vi "Gergberg Main.vi"() -> ()   [LabVIEW 2012, in "LightPipes.lvlib"]
uses:
  LightPipes.lvlib
panel:
  out "n_grid":i32=400
  in  "Number of Iteration":i32=20
  in  "MF Crop Size":i32=1000
  out "MF Interp Size":cluster{"x":i32, "y":i32}={"x"=1000, "y"=1000}
  out "MF Interped Pic":T1(plugin-control)
  in  "MF Interp Ratio":dbl=1.0
  in  "Mid Field":path=path "E:/MidfieldFarfieldForAaron/005778 2013-02-12/OSP Midfield.png"
  out "FF Interp Size":cluster{"x":i32, "y":i32}={"x"=1000, "y"=1000}
  out "FF Interp Pic":T1(plugin-control)
  in  "FF Crop Size":i32=400
  in  "FF Interp Ratio":dbl=2.5
  in  "Far Field":path=path "E:/MidfieldFarfieldForAaron/005778 2013-02-12/OSP FF.png"
  # "Far Field"
  # "Mid Field"
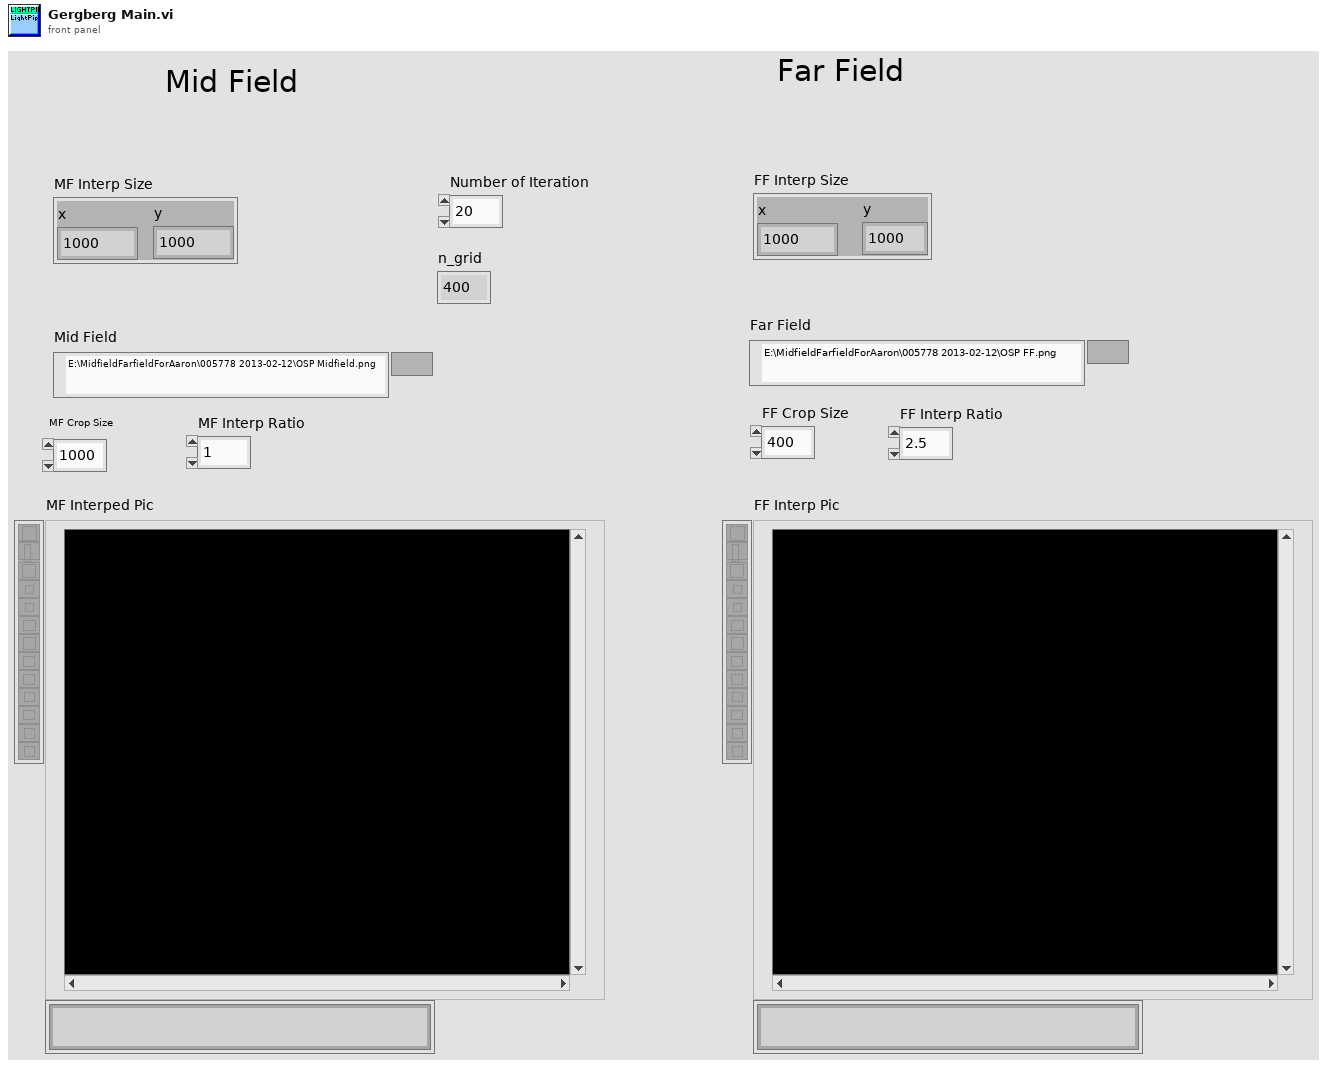
[diagram p1: front panel]
types:
  T1 = typedef "IMAQ Image.ctl" = refnum<image>
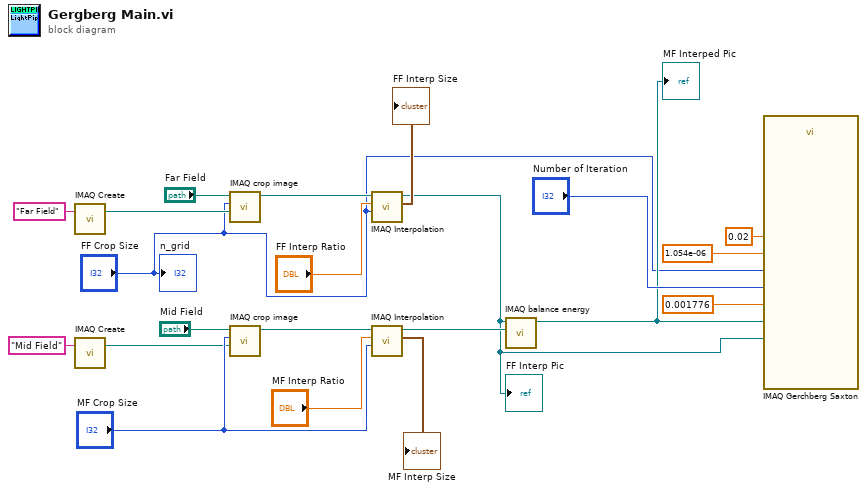
[diagram p0: block diagram]
diagram:
  n1 = call "IMAQ Create"("Image Name"="Far Field") -> ("New Image"=w14:T1)  [unwired: 4 in, 1 out]
  n2 = call "IMAQ Create"("Image Name"="Mid Field") -> ("New Image"=w15:T1)  [unwired: 4 in, 1 out]
  n3 = call "IMAQ crop image.vi"("Image"=w14, "Square Image Size"="FF Crop Size", "Path to PNG file"="Far Field") -> ("Cropped"=w12:T1)  [unwired: 8 in]
  n4 = call "IMAQ crop image.vi"("Image"=w15, "Square Image Size"="MF Crop Size", "Path to PNG file"="Mid Field") -> ("Cropped"=w13:T1)  [unwired: 8 in]
  n5 = call "IMAQ Interpolation.vi"("Image Size"="FF Crop Size", "Ratio"="FF Interp Ratio", "Image In"=w12) -> ("Interpolated Image Size"=→"FF Interp Size":cluster{"x":i32, "y":i32}, "Interpolated Image"=w5:T1)  [unwired: 7 in]
  "FF Interp Pic" <- w5
  n6 = call "IMAQ Interpolation.vi"("Image Size"="MF Crop Size", "Ratio"="MF Interp Ratio", "Image In"=w13) -> ("Interpolated Image Size"=→"MF Interp Size":cluster{"x":i32, "y":i32}, "Interpolated Image"=w6:T1)  [unwired: 7 in]
  n7 = call "IMAQ balance energy.vi"("Image B"=w6, "Image  A"=w5) -> ("Image"=w4:T1)  [unwired: 9 in]
  "MF Interped Pic" <- w4
  n8 = call "IMAQ Gerchberg Saxton.vi"("lambda"=1.054e-06, "forward distance"=0.02, "size_grid"=0.001776, "Number of Iteration"="Number of Iteration", "n_grid"="FF Crop Size", "Target"=w5, "Source"=w4) -> ()  [unwired: 3 in, 2 out]
  "n_grid" <- "FF Crop Size"
